vi "io_attr_write.vi"(7 "Attribute":T1={"Identifier"="", "Descriptive Name"="", "Data Type"=enum."Integer 32", "Command"="", "Access"=enum."Read/Write", "Range Table"="", "Read Callback"="", "Write Callback"="", "Supported Models"="", "Instrument Options"="", "Index"=0, "OPC Wait"=FALSE, "No Status Check"=FALSE, "Cache Only"=FALSE}, 8 "error in":errorcluster caption="error in (no error)", 10 "write buffer":string, 11 "VISA resource name":refnum<visa-resource-name>) -> (0 "error out":errorcluster, 3 "VISA resource name out":refnum<visa-resource-name>)   [LabVIEW 2022 SP3, in "hmp4000_rsidr_core.lvlib"]
uses:
  hmp4000_rsidr_core.lvlib
  type_Attribute.ctl
  type_Attribute_Data_Type.ctl
  type_ReadWriteAccess.ctl
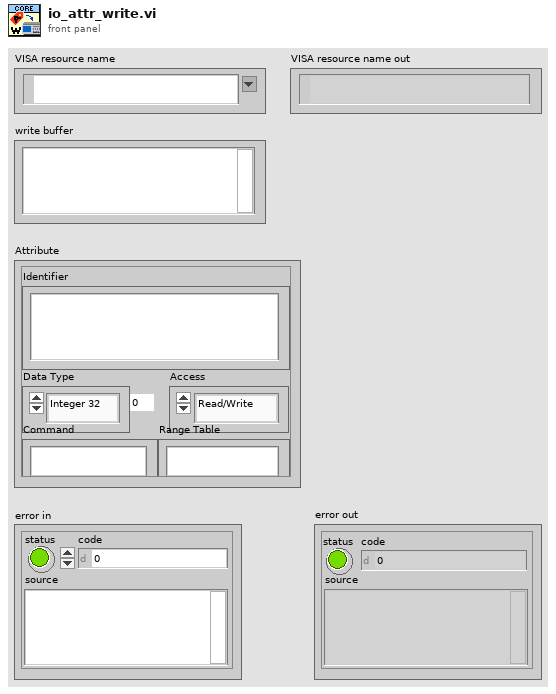
[diagram p1: front panel]
types:
  T1 = typedef "hmp4000_rsidr_core.lvlib/type_Attribute.ctl" = cluster{"Identifier":string, "Descriptive Name":string, "Data Type":T2, "Command":string, "Access":T3, "Range Table":string, "Read Callback":string, "Write Callback":string, "Supported Models":string, "Instrument Options":string, "Index":i32, "OPC Wait":bool, "No Status Check":bool, "Cache Only":bool}
  T2 = typedef "hmp4000_rsidr_core.lvlib/type_Attribute_Data_Type.ctl" = enum16{"Integer 32", "Double", "String", "Boolean", "None", "Integer 64", "RawString"}
  T3 = typedef "hmp4000_rsidr_core.lvlib/type_ReadWriteAccess.ctl" = enum16{"Read Only", "Write Only", "Read/Write"}
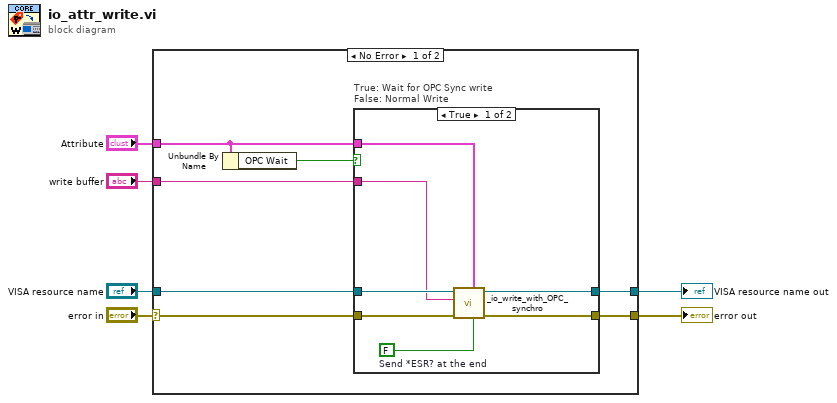
[diagram p0: block diagram]
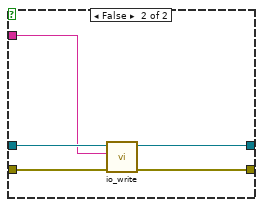
[diagram p2: hidden frame]
diagram:
  n1 = case shown="No Error" "error in" {
    selector: "error in" -> [w7 w27]
    tunnel: "VISA resource name" -> [w8 w26]
    tunnel: [w13 w27] -> w6
    tunnel: [w12 w26] -> w5
    tunnel: "Attribute" -> [w11 _]
    tunnel: "write buffer" -> [w10 _]
    frame No Error {
      n2 = Unbundle By Name(w11) -> ("OPC Wait"=w9:bool)
      n3 = case "True: Wait for OPC Sync write\nFalse: Normal Write" shown="True" w9 {
        tunnel: [w18 w23] -> w13
        tunnel: [w17 w22] -> w12
        tunnel: w7 -> [w20 w25]
        tunnel: w8 -> [w19 w24]
        tunnel: w11 -> [w15 _]
        tunnel: w10 -> [w16 w21]
        frame True {
          w14 = FALSE  # Send *ESR? at the end
          n4 = call "_io_write_with_OPC_synchro.vi"("Send *ESR? at the end (T)"=w14, "Attribute"=w15, "error in"=w20, "Write Command"=w16, "VISA resource name"=w19) -> ("error out"=w18:errorcluster, "VISA resource name out"=w17:refnum<visa-resource-name>)  [unwired: 4 in, 1 out]
        }
        frame False {
          n5 = call "io_write.vi"("error in"=w25, "write buffer"=w21, "VISA resource name"=w24) -> ("error out"=w23:errorcluster, "VISA resource name out"=w22:refnum<visa-resource-name>)  [unwired: 7 in]
        }
      }
    }
    frame Error {
    }
  }
  "VISA resource name out" <- w5
  "error out" <- w6
